vi "CaculateChord.vi"(0 "光斑横向像素":dbl, 5 "光斑纵向像素":dbl, 7 "当前距离":dbl, 9 "x轴角分辨":dbl, 11 "y轴角分辨":dbl) -> (6 "X轴弦长":dbl, 10 "Y轴弦长":dbl)   [LabVIEW 2018]
panel:
  # "从角度和距离计算当前圆的弦长"
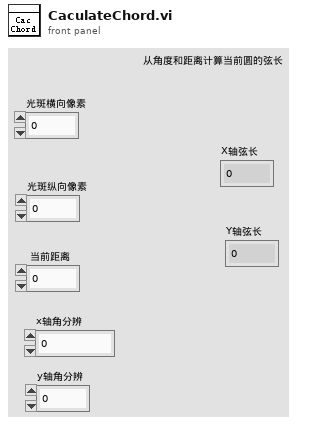
[diagram p1: front panel]
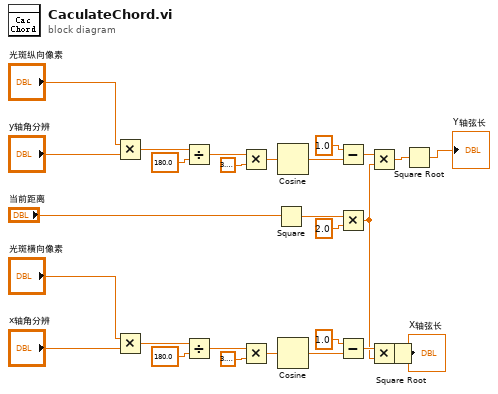
[diagram p0: block diagram]
diagram:
  n1 = Multiply(x="光斑纵向像素", y="y轴角分辨") -> (x*y=w11:dbl)
  n2 = Multiply(x="光斑横向像素", y="x轴角分辨") -> (x*y=w18:dbl)
  n3 = Divide(x=w11, y=180.0) -> (x/y=w13:dbl)
  n4 = Divide(x=w18, y=180.0) -> (x/y=w16:dbl)
  n5 = Multiply(x=w13, y=3.141592653589793) -> (x*y=w7:dbl)
  n6 = Multiply(x=w16, y=3.141592653589793) -> (x*y=w10:dbl)
  n7 = Square(x="当前距离") -> (x^2=w23:dbl)
  n8 = Cosine(x=w7) -> (cos(x)=w9:dbl)
  n9 = Cosine(x=w10) -> (cos(x)=w21:dbl)
  n10 = Subtract(x=1.0, y=w9) -> (x-y=w4:dbl)
  n11 = Multiply(x=w23, y=2.0) -> (x*y=w6:dbl)
  n12 = Subtract(x=1.0, y=w21) -> (x-y=w19:dbl)
  n13 = Multiply(x=w4, y=w6) -> (x*y=w3:dbl)
  n14 = Multiply(x=w19, y=w6) -> (x*y=w5:dbl)
  n15 = Square Root(x=w5) -> (sqrt(x)=→"X轴弦长":dbl)
  n16 = Square Root(x=w3) -> (sqrt(x)=→"Y轴弦长":dbl)
